vi "Loop_HW Motor.vi"() -> ()   [LabVIEW 2017, in "Hopper System.lvlib"]
uses:
  Hopper System.lvlib
  <vilib>/Rock Robotics/WPI/MotorControl/WPI_MotorControlDeviceRef.ctl
  <vilib>/Rock Robotics/WPI/MotorControl/WPI_MotorControlType.ctl
  <vilib>/Rock Robotics/SystemInterfaces/DIO/FPGA_DIOPWMChannel.ctl
  <vilib>/Rock Robotics/WPI/PWM/WPI_PWMDeadband.ctl
  <vilib>/Rock Robotics/SystemInterfaces/DIO/FPGA_DIOChannel.ctl
  Globals/Global_HW_Address_Assignments.vi
  Globals/Global_STOP.vi
  Global_SM_Data Out.vi
panel:
  out "Inner Output":dbl
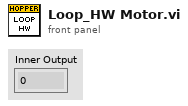
[diagram p1: front panel]
types:
  T1 = typedef "WPI_MotorControlDeviceRef.ctl" = cluster{"DeviceStatus":errorcluster, "Type":T2, "PWM":cluster{"PWM Channel":T3, "DeadBand":T4}, "CAN":cluster{"Device Number":u8, "SetOutput VI Ref":variant, "GetOutput VI Ref":variant, "Enable VI Ref":variant, "Disable VI Ref":variant, "Data":variant}, "Invert":bool, "DIO PWM":cluster{"PWM \"Enable\" Channel":T3, "DIOChannel":T5, "PWM Rate":dbl}}
  T2 = typedef "WPI_MotorControlType.ctl" = enum16{"PWM", "CAN", "DIO PWM"}
  T3 = typedef "FPGA_DIOPWMChannel.ctl" = enum8{"PWM 0", "PWM 1", "PWM 2", "PWM 3", "PWM 4", "PWM 5", "PWM 6", "PWM 7", "PWM 8", "PWM 9", "PWM MXP 0", "PWM MXP 1", "PWM MXP 2", "PWM MXP 3", "PWM MXP 4", "PWM MXP 5", "PWM MXP 6", "PWM MXP 7", "PWM MXP 8", "PWM MXP 9", "Invalid"}
  T4 = typedef "WPI_PWMDeadband.ctl" = cluster{"Name":string, "maxPositivePwm":i32, "minPositivePwm":i32, "centerPwm":i32, "maxNegativePwm":i32, "minNegativePwm":i32, "angularRange":u16}
  T5 = typedef "FPGA_DIOChannel.ctl" = enum8{"DIO 0", "DIO 1", "DIO 2", "DIO 3", "DIO 4", "DIO 5", "DIO 6", "DIO 7", "DIO 8", "DIO 9", "DIO MXP 0", "DIO MXP 1", "DIO MXP 2", "DIO MXP 3", "DIO MXP 4", "DIO MXP 5", "DIO MXP 6", "DIO MXP 7", "DIO MXP 8", "DIO MXP 9", "DIO MXP 10", "DIO MXP 11", "DIO MXP 12", "DIO MXP 13", "DIO MXP 14", "DIO MXP 15", "SPI Port CS1", "SPI Port CS2", "SPI Port CS3", "SPI Port MISO", "SPI Port MOSI", "Invalid"}
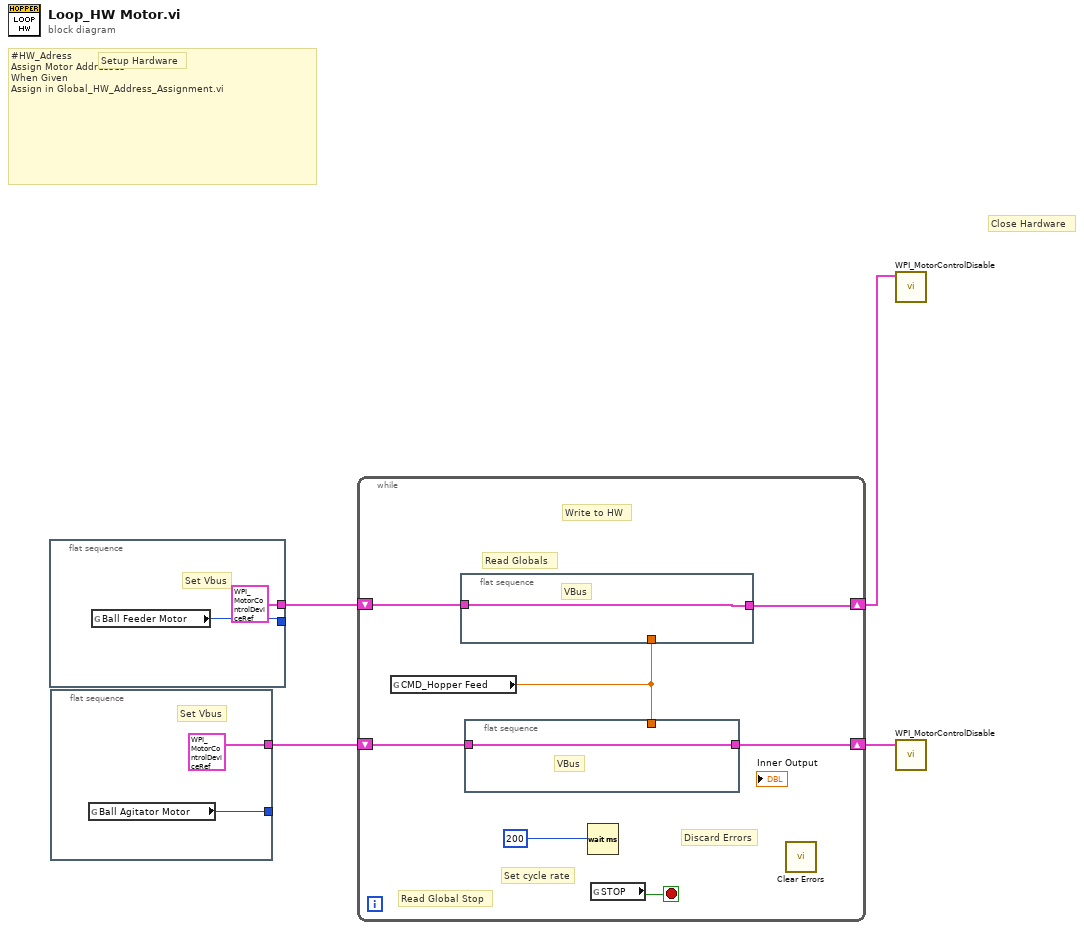
[diagram p0: block diagram]
diagram:
  # "#HW_Adress\nAssign Motor Addresses\nWhen Given\nAssign in Global_HW_Address_Assignment.vi"
  # "Close Hardware"
  # "Setup Hardware"
  n1 = flat-sequence {
    tunnel: [T1 {"DeviceStatus"={"status"=FALSE, "code"=0, "source"=""}, "Type"=enum."PWM", "PWM"={"PWM Channel"=enum."Invalid", "DeadBand"={"Name"="", "maxPositivePwm"=0, "minPositivePwm"=0, "centerPwm"=0, "maxNegativePwm"=0, "minNegativePwm"=0, "angularRange"=0}}, "CAN"={"Device Number"=0, "SetOutput VI Ref"=variant, "GetOutput VI Ref"=variant, "Enable VI Ref"=variant, "Disable VI Ref"=variant, "Data"=variant}, "Invert"=FALSE, "DIO PWM"={"PWM \"Enable\" Channel"=enum."Invalid", "DIOChannel"=enum."Invalid", "PWM Rate"=0.0}} ("CAN Talon SRX Ref")] -> w2
    tunnel: [w5] -> _
    frame #0 {
      # "Set Vbus"
      n2 = global read "Global_HW_Address_Assignments.vi" "Ball Feeder Motor"() -> (w5:u8)
    }
  }
  n3 = flat-sequence {
    tunnel: [T1 {"DeviceStatus"={"status"=FALSE, "code"=0, "source"=""}, "Type"=enum."PWM", "PWM"={"PWM Channel"=enum."Invalid", "DeadBand"={"Name"="", "maxPositivePwm"=0, "minPositivePwm"=0, "centerPwm"=0, "maxNegativePwm"=0, "minNegativePwm"=0, "angularRange"=0}}, "CAN"={"Device Number"=0, "SetOutput VI Ref"=variant, "GetOutput VI Ref"=variant, "Enable VI Ref"=variant, "Disable VI Ref"=variant, "Data"=variant}, "Invert"=FALSE, "DIO PWM"={"PWM \"Enable\" Channel"=enum."Invalid", "DIOChannel"=enum."Invalid", "PWM Rate"=0.0}} ("CAN Talon SRX Ref")] -> w1
    tunnel: [w7] -> _
    frame #0 {
      # "Set Vbus"
      n4 = global read "Global_HW_Address_Assignments.vi" "Ball Agitator Motor"() -> (w7:u8)
    }
  }
  n5 = while {
    shift-right: [w13] -> w4
    shift-left: w2 -> [w11]
    shift-right: [w9] -> w3
    shift-left: w1 -> [w12]
    stop <- w15 stop-if-true
    # "Write to HW"
    # "Discard Errors"
    # "Read Globals"
    # "Read Global Stop"
    # "Set cycle rate"
    n6 = global read "Global_SM_Data Out.vi" "CMD_Hopper Feed"() -> (w10:dbl)
    n7 = flat-sequence {
      tunnel: [w17] -> w13
      tunnel: w11 -> [w17]
      tunnel: w10 -> [_]
      frame #0 {
        # "VBus"
      }
    }
    n8 = flat-sequence {
      tunnel: w12 -> [w16]
      tunnel: w10 -> [_]
      tunnel: [w16] -> w9
      frame #0 {
        # "VBus"
      }
    }
    n9 = Wait (ms)(milliseconds to wait=u32 200) -> ()  [unwired: 1 out]
    n10 = global read "Global_STOP.vi" "STOP"() -> (w15:bool)
    n11 = call <vilib>:"Clear Errors.vi"() -> ()  [unwired: 6 in, 2 out]
  }
  n12 = call <vilib>:"WPI_MotorControlDisable.vi"("MotorControlDevRef"=w4) -> ()  [unwired: 9 in, 2 out]
  n13 = call <vilib>:"WPI_MotorControlDisable.vi"("MotorControlDevRef"=w3) -> ()  [unwired: 9 in, 2 out]
